vi "cmdJsonToArrayId.vi"(8 "error in":errorcluster, 9 "Control Data":T1, 10 "StreamCluster":T2={"DAQ"={"ManagmentRate_Hz"=1, "StreamRate_Hz"=50, "StreamRate_ms"=20, "ManagmentRate_ms"=1000, "refDesArray"=[]}, "Modules"=[]}, 11 "JSON in":string) -> (0 "error out":errorcluster, 3 "Control Data":T1)   [LabVIEW 2024]
uses:
  Control/StreamCluster_TypeDef.ctl
  Control/Control Data Constant.ctl
  745aa498-3cb0-4bfa-89e2-c2c9beed54ef.vi
  c49e8bee-f697-436e-a8eb-f13d28c7991d.vi
  <vilib>/JDP Science/JSONtext/Find Item.vi
  <vilib>/JDP Science/JSONtext/Next JSON Value.vi
  <vilib>/JDP Science/JSONtext/String Subset.vi
  <vilib>/JDP Science/JSONtext/Parsing/Advance past next JSON Value (inlined COPY).vi
  <vilib>/JDP Science/JSONtext/Parsing/Advance past whitespace.vi
  <vilib>/JDP Science/JSONtext/Parsing/Advance past String.vi
  <vilib>/JDP Science/JSONtext/Parsing/Advance past Number.vi
  <vilib>/JDP Science/JSONtext/Parsing/Advance past Line Ending.vi
  <vilib>/JDP Science/JSONtext/Parsing/Parse Full Path or Item Name.vi
  <vilib>/JDP Science/JSONtext/Parsing/Advance past Array.vi
  <vilib>/JDP Science/JSONtext/Parsing/Advance past Object.vi
  <vilib>/JDP Science/JSONtext/support/Error Cluster From Code.vi
  <vilib>/JDP Science/JSONtext/Offset/Find Item Locations by Path.vi
  <vilib>/JDP Science/JSONtext/JSON text to Variant.vi
  <vilib>/JDP Science/JSONtext/LVClass Serializer/JSONtext LVClass Serializer.lvclass
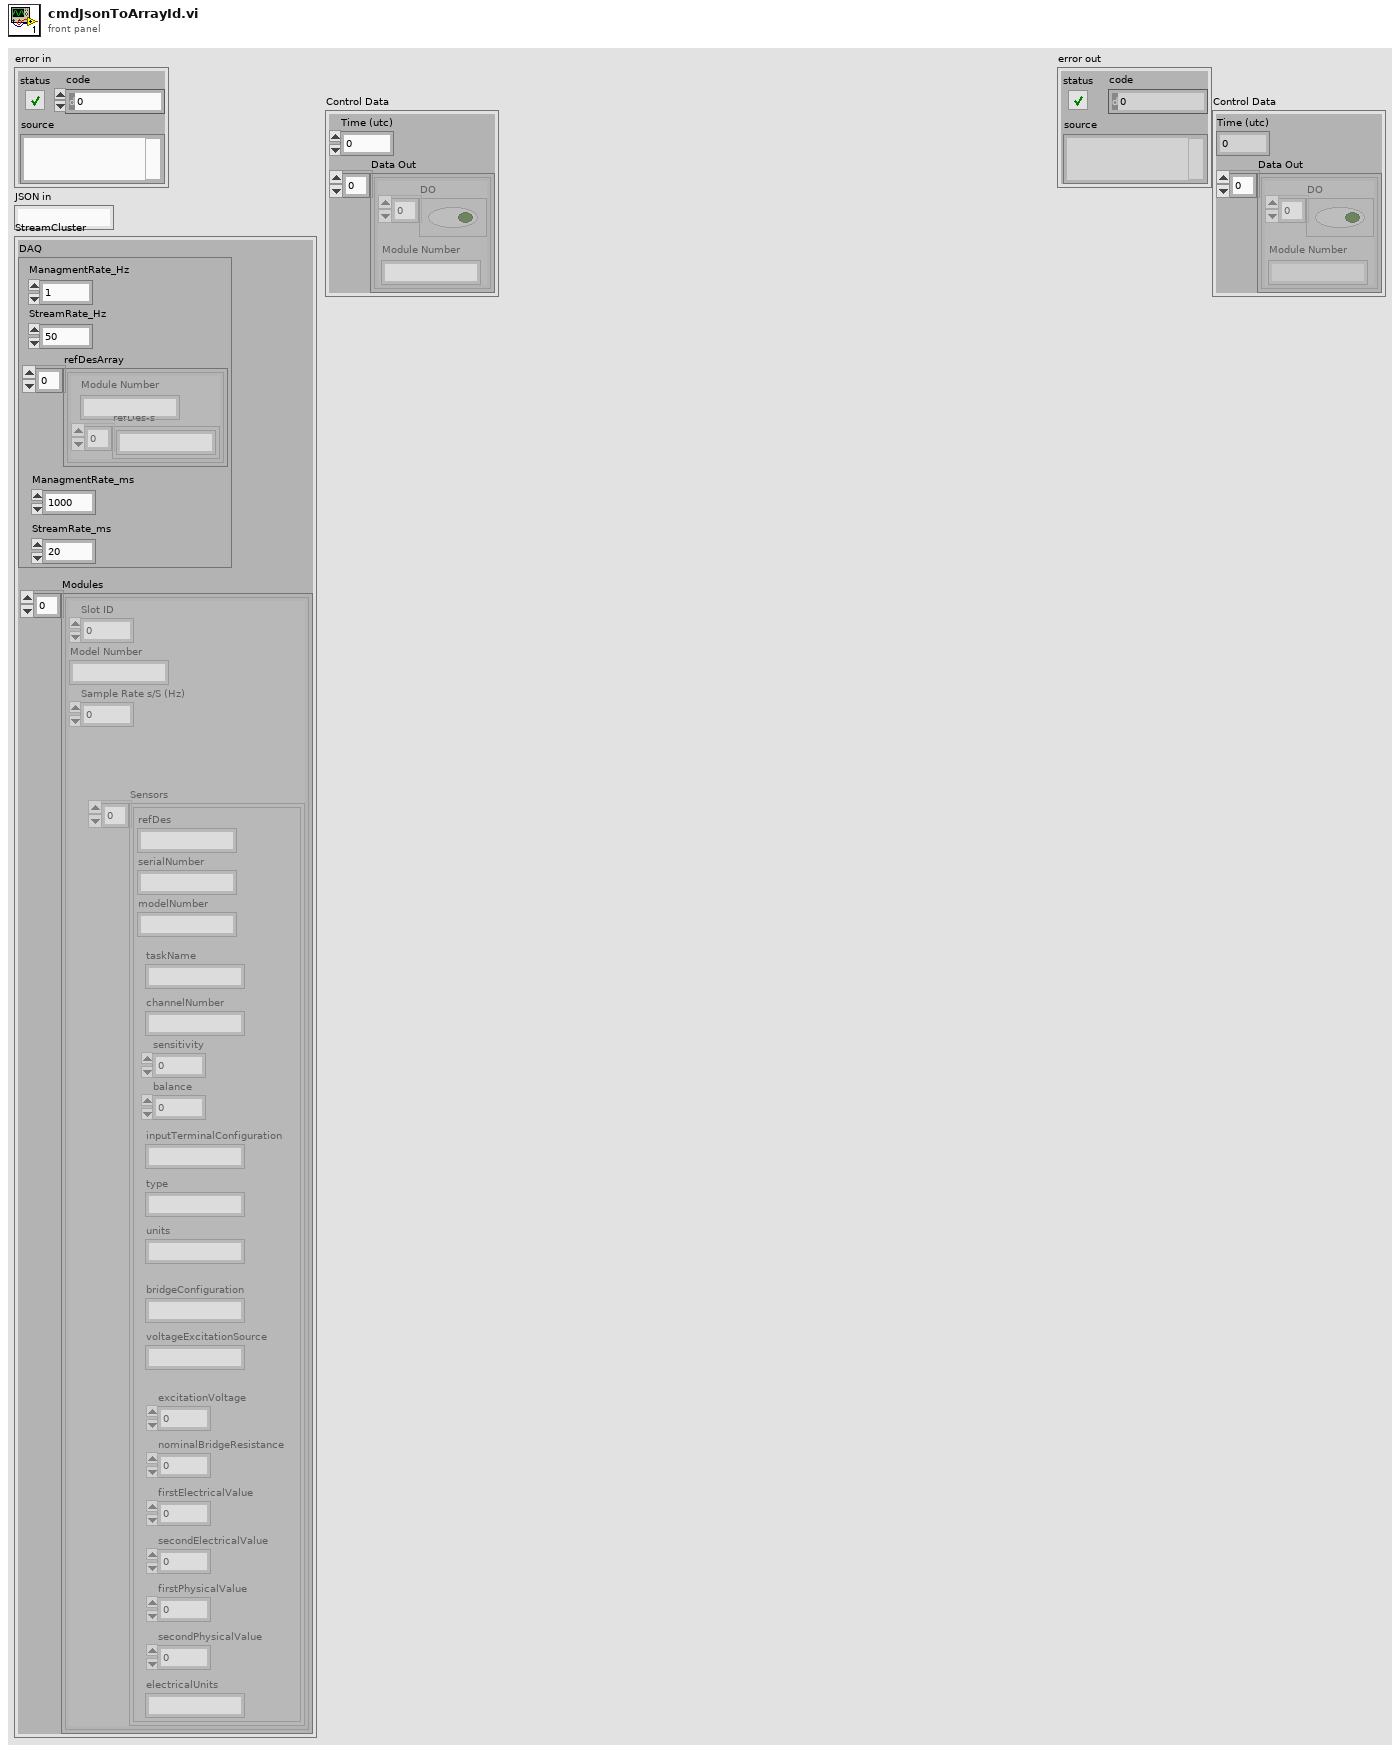
[diagram p1: front panel]
types:
  T1 = typedef "Control Data Constant.ctl" = cluster{"Time (utc)":ext, "Data Out":cluster{"DO":bool[], "Module Number":string}[]}
  T2 = typedef "StreamCluster_TypeDef.ctl" = cluster{"DAQ":cluster{"ManagmentRate_Hz":i32, "StreamRate_Hz":i32, "StreamRate_ms":i32, "ManagmentRate_ms":i32, "refDesArray":cluster{"refDes-s":string[], "Module Number":string}[]}, "Modules":cluster{"Slot ID":i32, "Model Number":string, "Sample Rate s/S (Hz)":dbl, "Sensors":cluster{"refDes":string, "serialNumber":string, "modelNumber":string, "units":string, "balance":dbl, "sensitivity":dbl, "type":string, "inputTerminalConfiguration":string, "channelNumber":string, "taskName":string, "bridgeConfiguration":string, "excitationVoltage":dbl, "voltageExcitationSource":string, "nominalBridgeResistance":dbl, "firstElectricalValue":dbl, "secondElectricalValue":dbl, "firstPhysicalValue":dbl, "secondPhysicalValue":dbl, "electricalUnits":string}[]}[]}
  T3 = cluster{"refDes-s":string[], "Module Number":string}[]
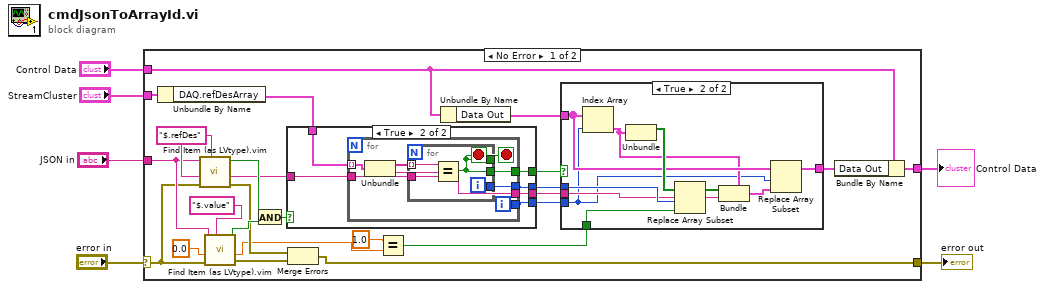
[diagram p0: block diagram]
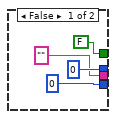
[diagram p3: hidden frame]
diagram:
  n1 = case shown="No Error" "error in" {
    selector: "error in" -> [w25 w66]
    tunnel: [w20 w66] -> w5
    tunnel: "JSON in" -> [w28 _]
    tunnel: "StreamCluster" -> [w24 _]
    tunnel: "Control Data" -> [w15 w65]
    tunnel: [w13 w65] -> w1
    frame No Error {
      w31 = "$.refDes" ("$Path or Item Name")
      n2 = Unbundle By Name(w24) -> ("DAQ.refDesArray"=w8:T3)
      n3 = call "Find Item (as LVtype).vim"("$Path or Item Name"=w31, "error in (no error)"=w25, "Data Type and Default Value"=w31, "JSON"=w28) -> ("error out"=w21:errorcluster, "Data"=w26:string, "Found"=w27:bool)  [unwired: 4 in, 1 out]
      n4 = call "Find Item (as LVtype).vim"("$Path or Item Name"="$.value", "error in (no error)"=w25, "Data Type and Default Value"=0.0, "JSON"=w28) -> ("error out"=w22:errorcluster, "Data"=w11:dbl, "Found"=w30:bool)  [unwired: 4 in, 1 out]
      n5 = And(x=w27, y=w30) -> (x .and. y?=w23:bool)
      n6 = case shown="True" w23 {
        tunnel: w26 -> [_ w52]
        tunnel: w8 -> [_ w51]
        tunnel: [0 w50] -> w18
        tunnel: [0 w49] -> w17
        tunnel: [FALSE w48] -> w19
        tunnel: ["" ("Module Number") w47] -> w7
        frame False {
        }
        frame True {
          n7 = for {
            tunnel: w52 -> [w58]
            tunnel: w51 -> [w60] mode=indexing
            tunnel: [w56] -> w48
            tunnel: [w55] -> w50
            tunnel: [w54] -> w49
            tunnel: [w53] -> w47
            i -> [w54]
            stop <- w57 stop-if-true
            n8 = Unbundle(w60) -> ("refDes-s"=w59:string[], "Module Number"=w53:string)
            n9 = for {
              tunnel: w59 -> [w64] mode=indexing
              tunnel: w58 -> [w63]
              tunnel: [w62] -> w57
              tunnel: [w62] -> w56
              tunnel: [w61] -> w55
              i -> [w61]
              stop <- w62 stop-if-true
              n10 = Equal?(x=w64, y=w63) -> (x = y?=w62:bool)
            }
          }
        }
      }
      n11 = Merge Errors(w21, w22) -> (w20:errorcluster)
      n12 = Equal?(x=1.0, y=w11) -> (x = y?=w9:bool)
      n13 = Unbundle By Name(w15) -> ("Data Out"=w16:cluster{"DO":bool[], "Module Number":string}[])
      n14 = case shown="True" w19 {
        tunnel: w9 -> [_ w41]
        tunnel: w16 -> [w32 w39]
        tunnel: w18 -> [_ w40]
        tunnel: w17 -> [_ w33]
        tunnel: [w32 w38] -> w14
        tunnel: w7 -> [_ w34]
        frame False {
        }
        frame True {
          n15 = Index Array(array=w39, index=w33) -> (element=w37:cluster{"DO":bool[], "Module Number":string})
          n16 = Unbundle(w37) -> ("DO"=w42:bool[])  [unwired: 1 out]
          n17 = Replace Array Subset(array=w42, new element=w41, index=w40) -> (w36:bool[])
          n18 = Bundle(cluster=w37, "DO"=w36, "Module Number"=w34) -> (w35:cluster{"DO":bool[], "Module Number":string})
          n19 = Replace Array Subset(array=w39, new element=w35, index=w33) -> (w38:cluster{"DO":bool[], "Module Number":string}[])
        }
      }
      n20 = Bundle By Name(cluster=w15, "Data Out"=w14) -> (w13:T1)
    }
    frame Error {
    }
  }
  "error out" <- w5
  "Control Data" <- w1
